vi "3D Pie Graph.vi"() -> ()   [LabVIEW 2023]
doc: "This VI shows how to use the 3D Pie Plot."
uses:
  <vilib>/Math Plots/3D Math Plots/3D Pie/3D Pie XCtrl/3D Pie.xctl
  <vilib>/Math Plots/3D Math Plots/3D Pie/3D Pie Datatype/Public/Plot Helper (Vector).vi
  <vilib>/Math Plots/3D Math Plots/3D Pie/3D Pie Datatype/3D Pie Datatype.lvclass
panel:
  out "3D Pie":refnum<class "3D Plot Datatype.lvclass">[](xcontrol)
  # "Overview: Demonstrates the Pie indicator from the Graph > 3D Graph palette.\nRequirements: LabVIEW Full Development System\nInstructions:\nRun the VI."
  # "Try the following operations on the graph:\n\n1. Click and drag the mouse within the graph to change the view direction.\n2. Press the Shift key and drag the mouse up to zoom in.\n3. Press the Shift key and drag the mouse down to zoom out.\n4. Right-click the graph and choose 3D Plot Properties to configure various properties related to the graph's appearance.\n5. Right-click the graph and select Export Image >Export to File.\n6. Change the colors and names of the plots in the Color Palette in the upper-right corner of the graph."
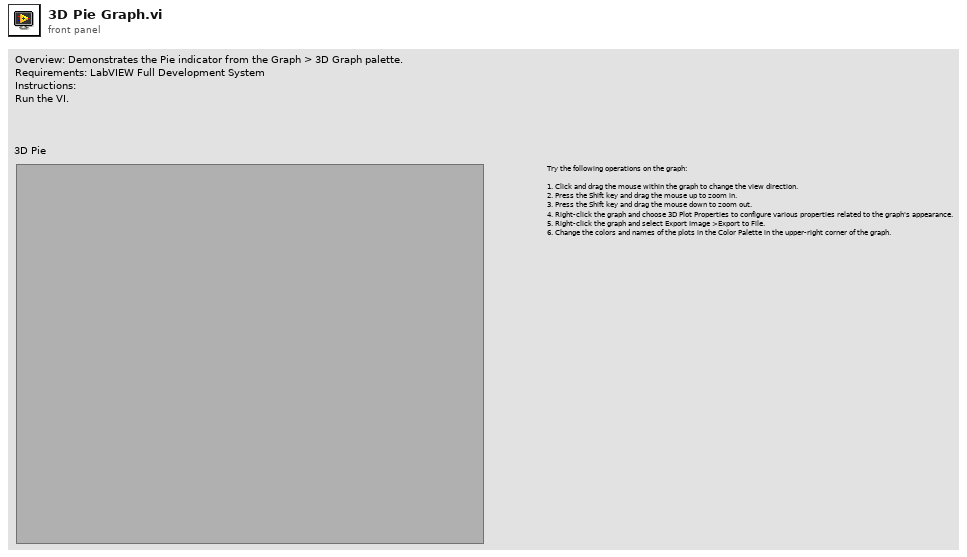
[diagram p1: front panel]
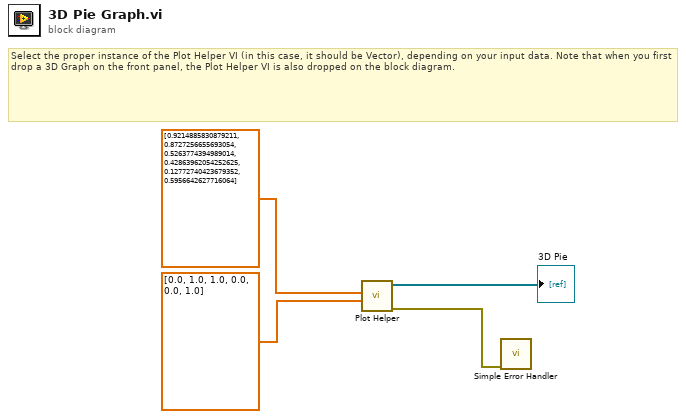
[diagram p0: block diagram]
diagram:
  # "Select the proper instance of the Plot Helper VI (in this case, it should be Vector), depending on your input data. Note that when you first drop a 3D Graph on the front panel, the Plot Helper VI is also dropped on the block diagram."
  n1 = call-poly <vilib>:"Plot Helper.vi"("offset vector"=sgl[] [0.0, 1.0, 1.0, 0.0, 0.0, 1.0], "x vector"=sgl[] [0.9214886, 0.87272567, 0.52637744, 0.42863962, 0.1277274, 0.59566426] ("offset vector")) -> ("error out"=w1:errorcluster, "3D Plot lvclass Array out"=→"3D Pie":refnum<class "3D Plot Datatype.lvclass">[])  [unwired: 2 in, 6 out]
  n2 = call <vilib>:"Simple Error Handler.vi"("error in (no error)"=w1) -> ()  [unwired: 4 in, 5 out]
